vi "Lockin_Vsg.vi"(8 "error in (no error)":errorcluster, 11 "Transport":refnum<class "SMO.Transport.lvclass">) -> (0 "error out":errorcluster, 3 "Transport out":refnum<class "SMO.Transport.lvclass">)   [LabVIEW 2019, in "SMO.Transport.lvclass"]
uses:
  SMO.Transport.lvclass
  <userlib>/LevyLab/Lockin-Multichannel/Instrument.Lockin/Instrument.Lockin.lvclass
  <userlib>/LevyLab/Instrument Framework/Instrument Types/Cryostat/Instrument.Cryostat.lvclass
  Control Experiment/Control Experiment.lvclass
  <userlib>/LevyLab/Krohn Hite 7008/Instrument.KH7008.lvclass
  Control Experiment/Typedefs/Instruments--cluster.ctl
  <userlib>/LevyLab/Instrument Framework/Instrument Types/VSource/Instrument.VSource.lvclass
  <userlib>/LevyLab/Instrument Framework/Instrument Types/VNA/Instrument.VNA.lvclass
  <userlib>/LevyLab/Instrument Framework/Instrument Types/Strain/Instrument.Strain.lvclass
  <userlib>/LevyLab/Instrument Framework/Instrument Types/CBridge/Instrument.CBridge.lvclass
  <userlib>/LevyLab/Instrument Framework/Instrument Types/Delay Line/Instrument.DelayLine.lvclass
panel:
  in  "Tab Control":enum32{"lockin/SG Control", "Data", "Other"}(tab)=enum."Data"
  out "elapsed time (s)":u32=1660
  in  "Side Gate Channel(s)":i32[](array[numeric])=[21]
  in  "Vmax (end)":dbl=5.0 format="%#_3p"
  in  "Vmin (start)":dbl=-5.0 format="%#_3p"
  in  "dV":dbl=0.025 format="%#_3p"
  in  "Experiment Comments":string="Vbg sweep from  0V to 100V to  -100V to 0V in steps of 0.5V\n\nstripe device:\n\nI+: 11,12,13, current mode, gain: 1000x, shunt resistor : 5kohm \nlead 12: Vac: 125uV, 7Hz, Vdc= 0mV\ndV1: 11-12 voltage mode, gain: 10x, shunt resistor : open \nVbg: 26, 1Gohm resistor\n\nhash device:\n\nI+: 16,17 current mode, gain: 1000x, shunt resistor : 5kohm \nlead 17: Vac:  5mV, 7Hz, Vdc= 0mV\n##lead 20, voltage mode, gain: 10x, shunt resistor : open \ndV1: 16-17 voltage mode, gain: 10x, shunt resistor : open \n##dV1: 16-20 voltage mode, gain: 10x, shunt resistor : open \nVbg: 26, 1Gohm resistor\n\nIn plane gates:\n3,8,15,21: 0V, 100Mohm resistors"
  in  "Experiment Folder":string="14- mega backgate sweep"
  out "T (mK)":dbl=0.001
  in  "wait after setting Vsg (ms)":u32=2000
  in  "Initial wait (ms)":u32=1000
  in  "Sweep":enum16{"Vsg", "Vbg"}(ring)
  in  "cycles (1,2,...)":i32=1 min=1 step=1
  in  "phase":dbl
  out "Field (T)":dbl=-0.0003 format="%#_13g"
  in  "function (ramp)":enum16{"Ramp", "Triangle", "Sine"}(ring)=enum."Triangle"
  in  "set \"Vsg\" to initial value?":bool
  out "time b/w points (ms)":u32=2066
  in  "stop":bool
  out "X Lockins":cluster{dbl[], dbl[]}[](graph)
  out "Y Lockins":cluster{dbl[], dbl[]}[](graph)
  out "G4T":cluster{dbl[], dbl[]}[](graph)
  # "*** These controls are only read if this VI is the top level. If is is called from Sweep Control then the folder and comments come from Sweep Control.vi ***"
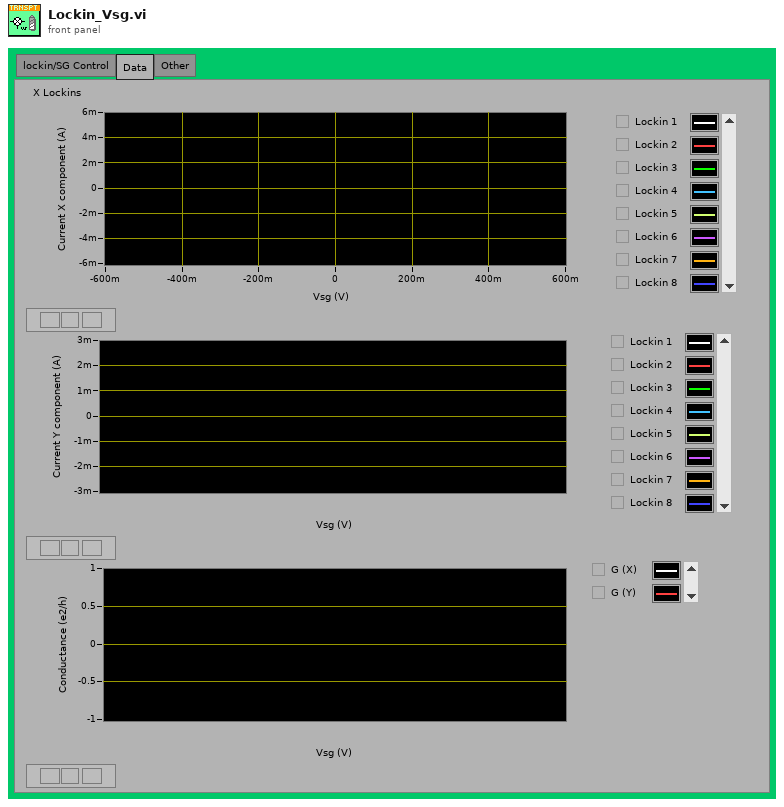
[diagram p1: front panel]
types:
  T1 = enum32{"Invalid", "Standard", "Closed", "Hidden", "Minimized", "Maximized"}
  T2 = enum32{"invalid app kind", "Development System", "Run Time System", "Student Edition", "Embedded LabVIEW", "Evaluation", "Custom"}
  T3 = typedef "Control Experiment.lvclass/Instruments--cluster.ctl" = cluster{"KH7008":refnum<class "Instrument.KH7008.lvclass">[], "Lockin":refnum<class "Instrument.Lockin.lvclass">, "Temperature":refnum<class "Instrument.Cryostat.lvclass">, "Magnet":refnum<class "Instrument.Cryostat.lvclass">, "Rotator":refnum<class "Instrument.Cryostat.lvclass">, "Level":refnum<class "Instrument.Cryostat.lvclass">, "Capacitance Bridge":refnum<class "Instrument.CBridge.lvclass">, "Delay Line":refnum<class "Instrument.DelayLine.lvclass">, "Strain Cell":refnum<class "Instrument.Strain.lvclass">, "VNA":refnum<class "Instrument.VNA.lvclass">, "Voltage Source":refnum<class "Instrument.VSource.lvclass">}
  T4 = cluster{"Core":cluster{"Current VI Reference":refnum<vi>, "Close Panel on Exit?":bool}, "Transport":refnum<class "SMO.Transport.lvclass">, "Control Experiment":refnum<class "Control Experiment.lvclass">, "Instruments":T3, "Sweep Values":dbl[], "Results (Dictionary)":cluster{"key":string, "value":dbl}[], "size":i32, "index":i32, "ms [0]":u32, "ms [i]":u32, "Execution:State":enum32{"Bad", "Idle", "Run top level", "Running"}}
  T5 = enum32{"Bad", "Idle", "Run top level", "Running"}
  T6 = cluster{"Current VI Reference":refnum<vi>, "Close Panel on Exit?":bool}
  T7 = cluster{"I-":i32, "I+":i32, "V1-":i32, "V1+":i32, "I2-":i32, "I2+":i32, "V2-":i32, "V2+":i32}
  T8 = typedef "Instrument.DAQ.lvclass/AO.Channel--Cluster--Array.ctl" = T9[]
  T9 = typedef "Instrument.DAQ.lvclass/AO.Channel--Cluster.ctl" = cluster{"Enable?":bool, "Channel":i32, "Amplitude":dbl, "Offset":dbl, "Frequency":dbl, "Phase":dbl, "Function":T10, "Sweeping?":bool}
  T10 = typedef "Instrument.DAQ.lvclass/AO.Channel.Function--Enum.ctl" = enum16{"Sine", "Triangle", "Square"}
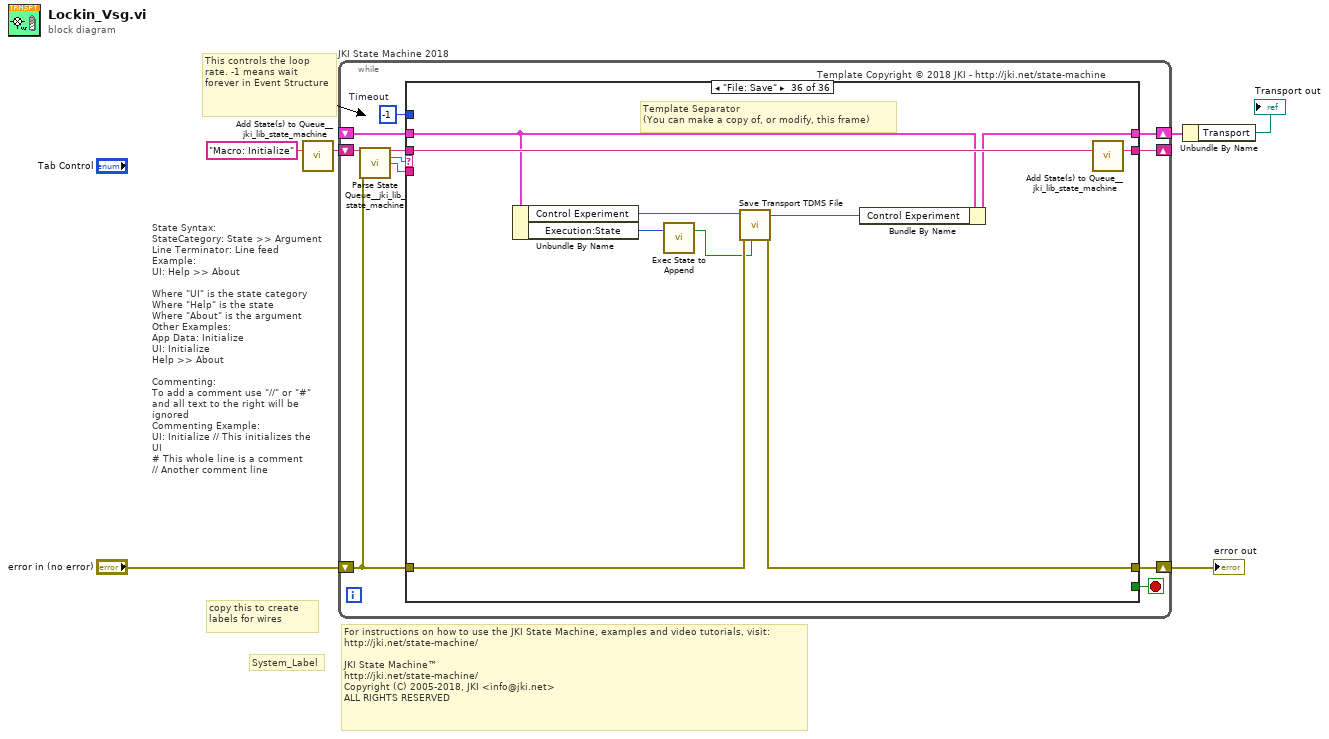
[diagram p0: block diagram]
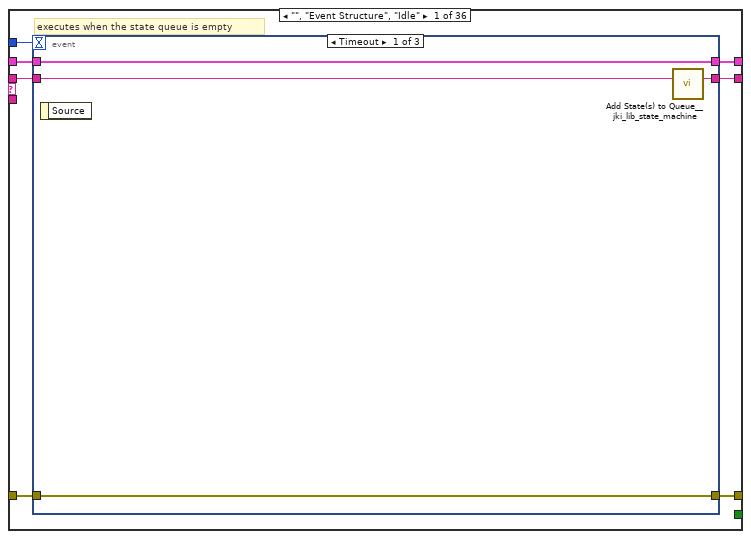
[diagram p2: hidden frame]
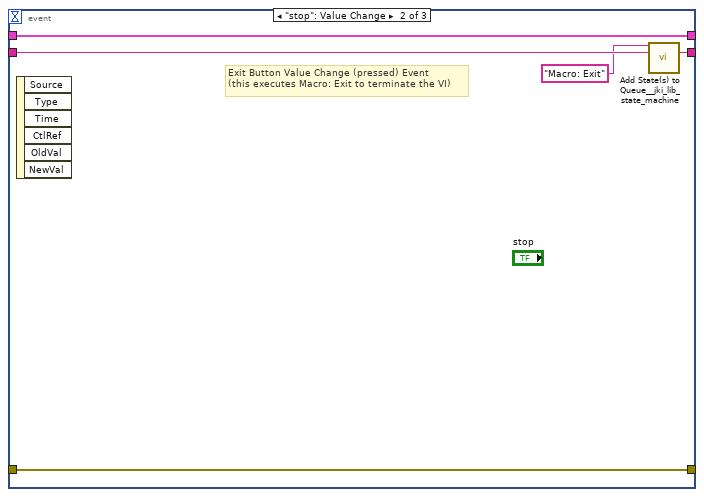
[diagram p3: hidden frame]
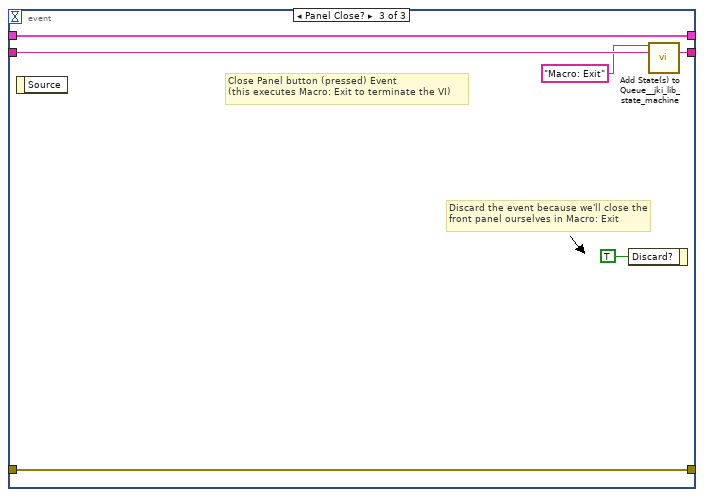
[diagram p4: hidden frame]
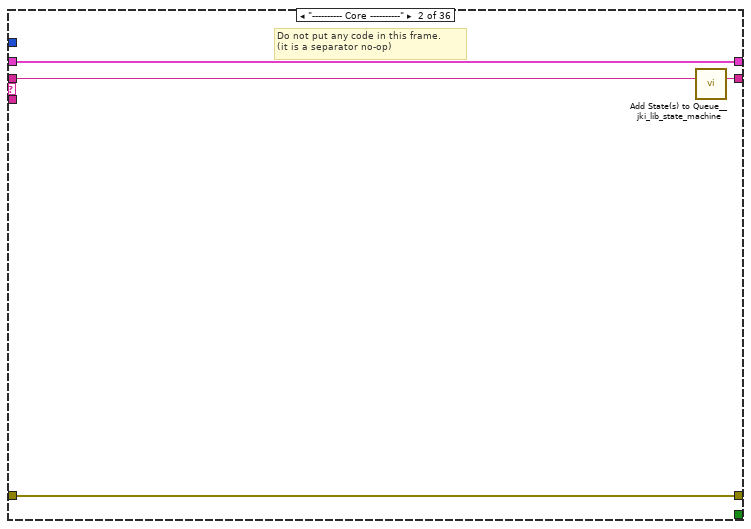
[diagram p5: hidden frame]
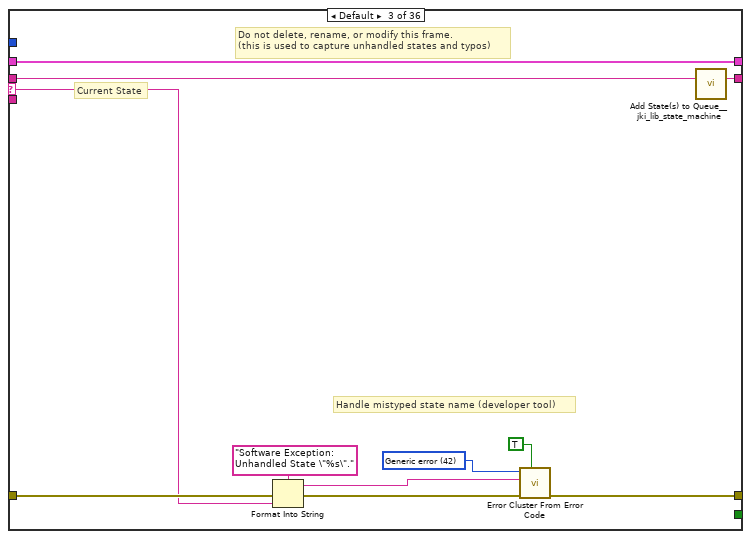
[diagram p6: hidden frame]
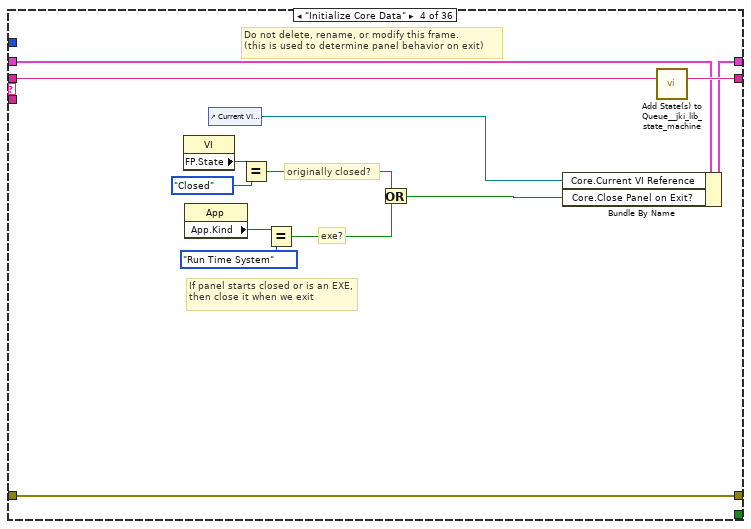
[diagram p7: hidden frame]
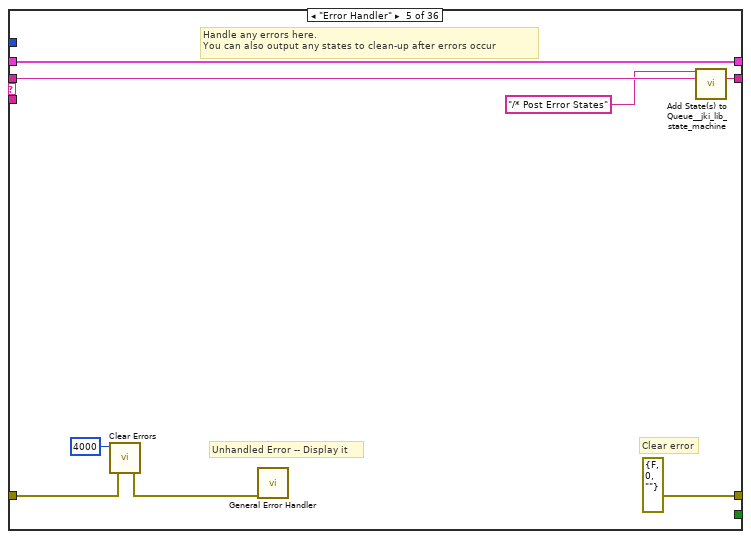
[diagram p8: hidden frame]
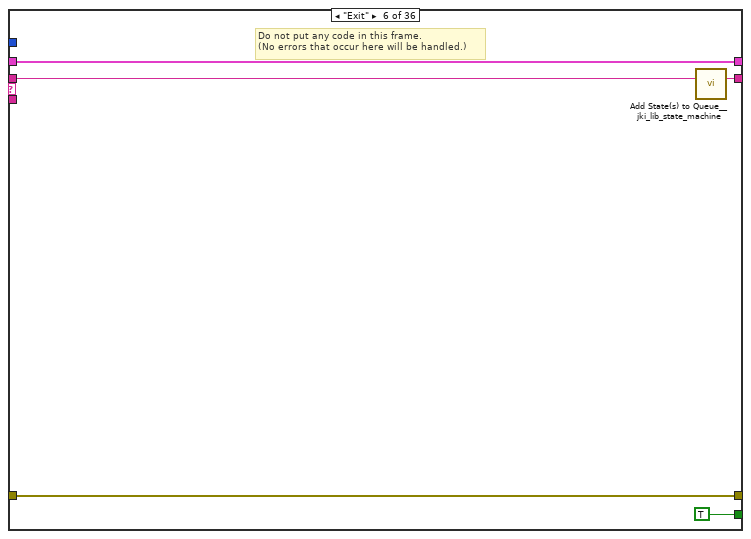
[diagram p9: hidden frame]
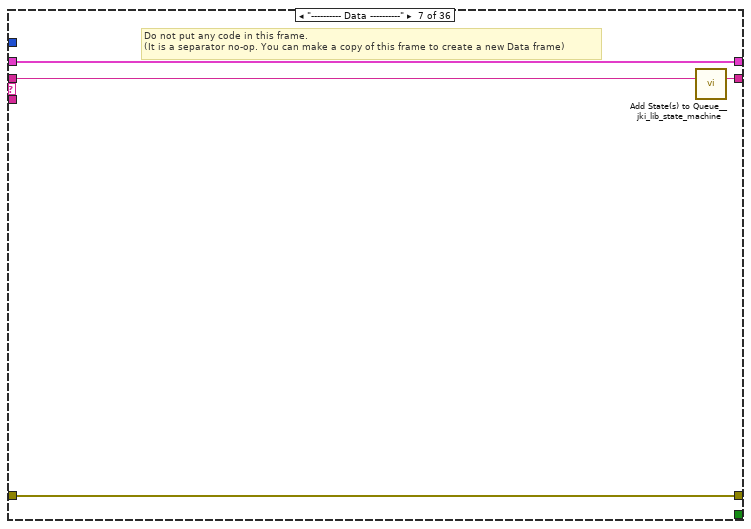
[diagram p10: hidden frame]
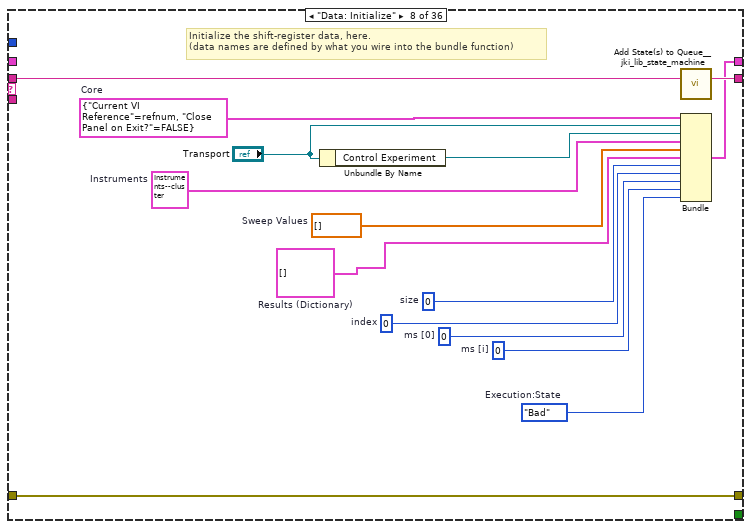
[diagram p11: hidden frame]
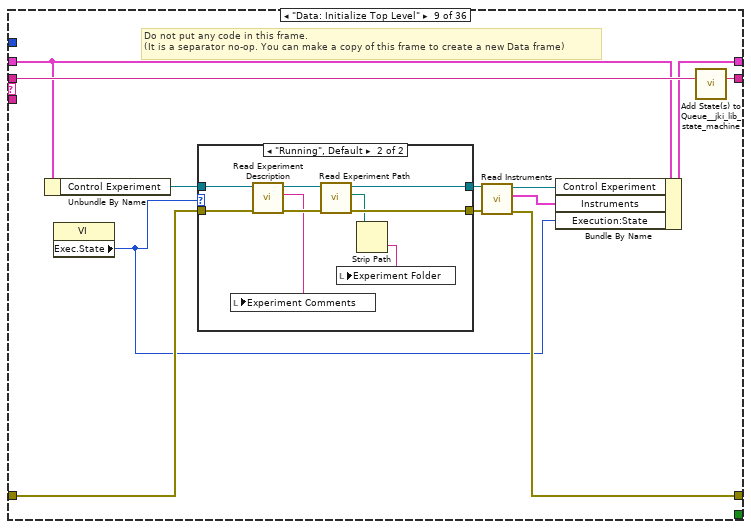
[diagram p12: hidden frame]
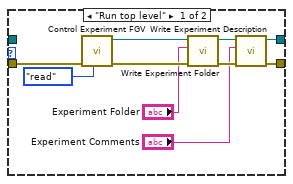
[diagram p13: hidden frame]
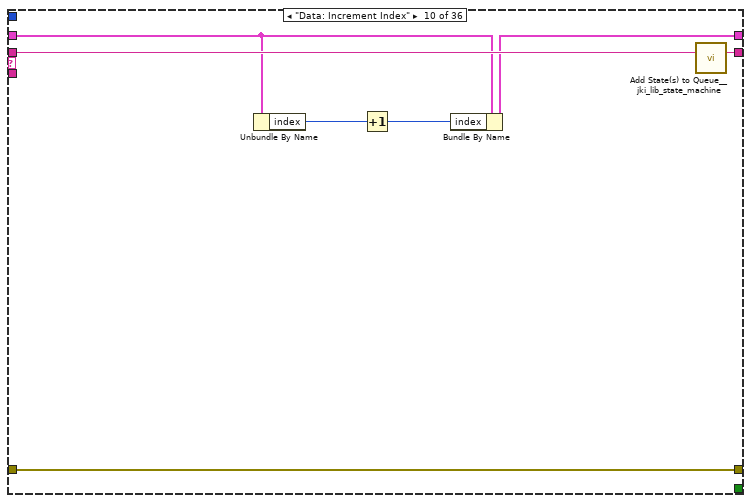
[diagram p14: hidden frame]
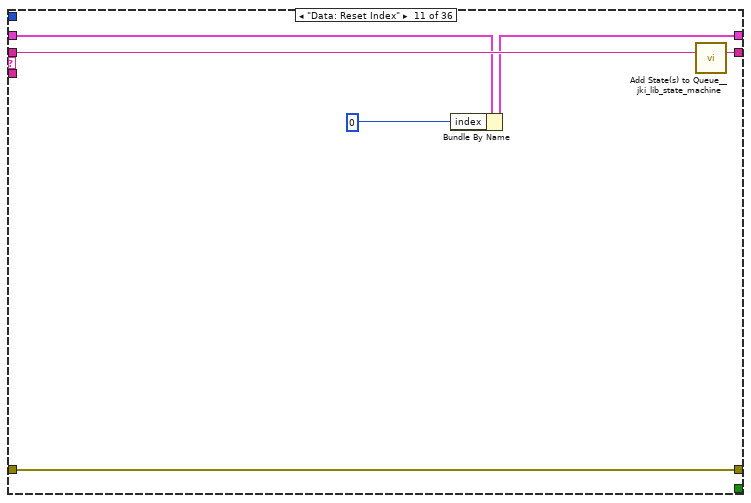
[diagram p15: hidden frame]
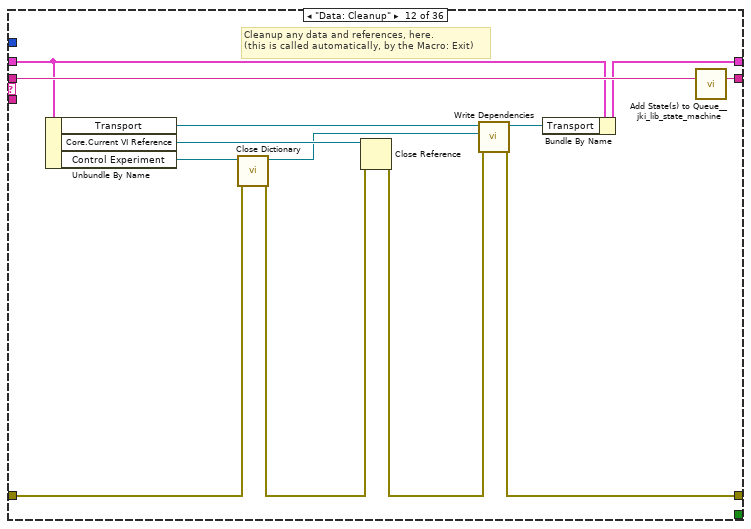
[diagram p16: hidden frame]
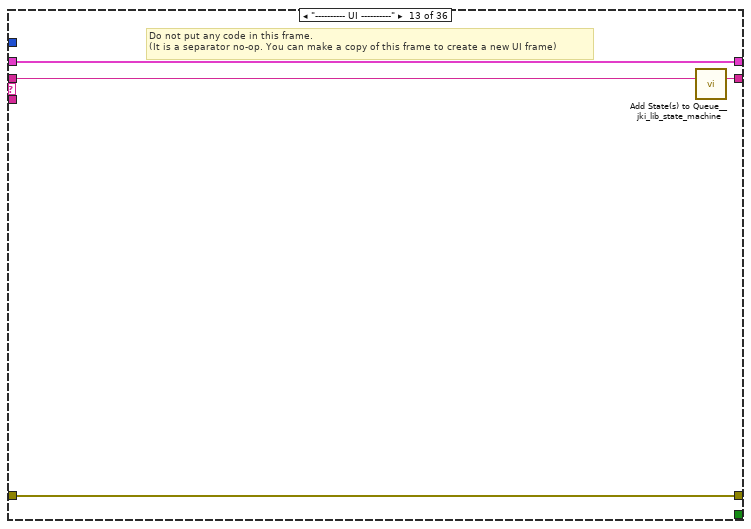
[diagram p17: hidden frame]
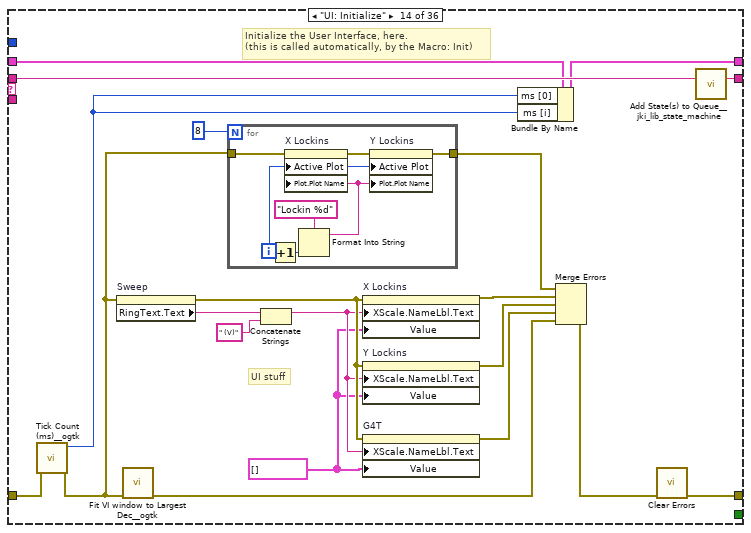
[diagram p18: hidden frame]
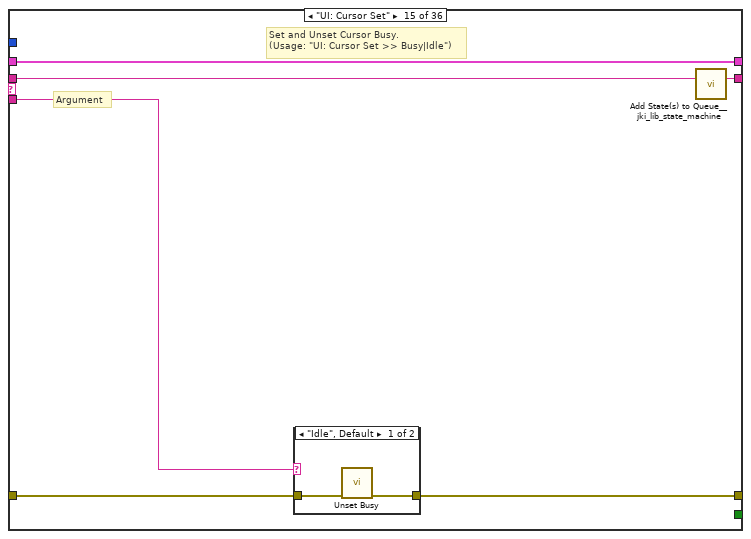
[diagram p19: hidden frame]
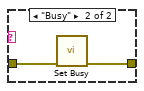
[diagram p20: hidden frame]
diagram:
  # "For instructions on how to use the JKI State Machine, examples and video tutorials, visit:\nhttp://jki.net/state-machine/\n\nJKI State Machine™\nhttp://jki.net/state-machine/\nCopyright (C) 2005-2018, JKI <info@jki.net>\nALL RIGHTS RESERVED"
  # "State Syntax:\nStateCategory: State >> Argument\nLine Terminator: Line feed\nExample:\nUI: Help >> About\n\nWhere \"UI\" is the state category\nWhere \"Help\" is the state\nWhere \"About\" is the argument\nOther Examples:\nApp Data: Initialize\nUI: Initialize\nHelp >> About\n\nCommenting:\nTo add a comment use \"//\" or \"#\" and all text to the right will be ignored\nCommenting Example:\nUI: Initialize // This initializes the UI\n# This whole line is a comment\n// Another comment line"
  # "copy this to create labels for wires"
  # "This controls the loop rate. -1 means wait forever in Event Structure"
  # "System_Label"
  n1 = call <vilib>:"Add State(s) to Queue__jki_lib_state_machine.vi"("State(s) in (\"\")"="Macro: Initialize") -> ("States Out"=w6:string)  [unwired: 14 in]
  n2 = while "JKI State Machine 2018" {
    shift-right: [w10] -> w4
    shift-left: _ -> [w9]
    shift-right: [w13] -> w2
    shift-left: "error in (no error)" -> [w7]
    shift-right: [w12] -> _
    shift-left: w6 -> [w14]
    stop <- w11 stop-if-true
    w8 = -1  # Timeout
    # "Template Copyright © 2018 JKI - http://jki.net/state-machine"
    n3 = call <vilib>:"Parse State Queue__jki_lib_state_machine.vi"("State Queue"=w14, "Error In (no error)"=w7) -> ("Remaining States"=w16:string, "Current State"=w17:string, "Arguments"=w15:string)  [unwired: 11 in]
    n4 = case shown="\"File: Save\"" w17 {
      selector: w17 -> [_ _ w44 _ _ _ _ _ _ _ _ _ _ _ _ _ _ _ _ _ _ _ _ _ _ _ _ _ _ _ _ _ _ _ _ _]
      tunnel: w16 -> [w24 w43 w48 w67 w75 w80 w84 w99 w111 w137 w143 w156 w160 w180 w193 w216 w229 w236 w305 w310 w332 w342 w346 w370 w382 w389 w401 w435 w447 w459 w471 w484 w511 w515 w519 w529]
      tunnel: w15 -> [_ _ _ _ _ _ _ _ _ _ _ _ _ _ w188 _ _ w230 _ _ _ _ _ _ _ _ _ _ _ _ _ _ _ _ _ _]
      tunnel: w9 -> [w22 w40 w46 w60 w72 w78 w81 _ w102 w131 w140 w145 w157 w164 w191 w199 w224 w232 w302 w308 w325 w339 w343 w358 w379 w385 w392 w432 w443 w456 w465 w479 w507 w512 w516 w523]
      tunnel: [w21 w41 w50 w64 errorcluster {"status"=FALSE, "code"=0, "source"=""} ("error out") w77 w82 w96 w103 w135 w141 w146 w158 w169 w189 w214 w218 w233 w303 w306 w330 w340 w344 w348 w380 w386 w395 w433 w439 w449 w461 w473 w502 w513 w517 w526] -> w13
      tunnel: w7 -> [w20 w41 w49 w64 w69 w77 w82 w96 w104 w135 w141 w152 w158 w166 w190 w214 w226 w234 w303 w306 w330 w340 w344 w355 w380 w387 w394 w433 w444 w454 w462 w482 w503 w513 w517 w525]
      tunnel: [w23 w42 w47 w66 w74 w79 w83 w98 w110 w136 w142 w155 w159 w179 w192 w215 w228 w235 w304 w309 w331 w341 w345 w369 w381 w388 w400 w434 w446 w458 w470 w483 w510 w514 w518 w528] -> w12
      tunnel: [_ _ _ _ _ TRUE _ _ _ _ _ _ _ _ _ _ _ _ _ _ _ _ _ _ _ _ _ _ _ _ _ _ _ _ _ _] -> w11
      tunnel: [w19 w40 w46 w65 w72 w78 w81 w97 w101 w134 w139 w149 w157 w163 w191 w199 w223 w232 w302 w308 w325 w339 w343 w361 w379 w385 w392 w432 w442 w455 w464 w480 w508 w512 w516 w522] -> w10
      tunnel: w8 -> [w18 _ _ _ _ _ _ _ _ _ _ _ _ _ _ _ _ _ _ _ _ _ _ _ _ _ _ _ _ _ _ _ _ _ _ _]
      frame "", "Event Structure", "Idle" {
        # "executes when the state queue is empty"
        n5 = event shown="[0] Timeout" {
          selector: _ -> [_ _ _]
          dyn-events: _ -> [_ _ _]
          timeout: w18 -> [_ _ _]
          tunnel: w24 -> [w28 w33 w39]
          tunnel: [w27 w32 w38] -> w23
          tunnel: w22 -> [w25 w30 w36]
          tunnel: [w26 w31 w37] -> w21
          tunnel: w20 -> [w26 w31 w37]
          tunnel: [w25 w30 w36] -> w19
          event Timeout {
            n6 = event-data() -> ()  [unwired: 1 in, 1 out]
            n7 = call <vilib>:"Add State(s) to Queue__jki_lib_state_machine.vi"("State(s) in (\"\")"=w28) -> ("States Out"=w27:string)  [unwired: 14 in]
          }
          event "stop": Value Change {
            # "Exit Button Value Change (pressed) Event\n(this executes Macro: Exit to terminate the VI)"
            n8 = event-data() -> ()  [unwired: 1 in, 6 out]
            n9 = call <vilib>:"Add State(s) to Queue__jki_lib_state_machine.vi"("State(s) in Front (\"\")"="Macro: Exit", "State(s) in (\"\")"=w33) -> ("States Out"=w32:string)  [unwired: 13 in]
          }
          event Panel Close? {
            # "Discard the event because we'll close the front panel ourselves in Macro: Exit"
            # "Close Panel button (pressed) Event\n(this executes Macro: Exit to terminate the VI)"
            n10 = event-data() -> ()  [unwired: 1 in, 1 out]
            n11 = event-data("Discard?"=TRUE) -> ()  [unwired: 1 in, 1 out]
            n12 = call <vilib>:"Add State(s) to Queue__jki_lib_state_machine.vi"("State(s) in Front (\"\")"="Macro: Exit", "State(s) in (\"\")"=w39) -> ("States Out"=w38:string)  [unwired: 13 in]
          }
        }
      }
      frame "---------- Core ----------" {
        # "Do not put any code in this frame.\n(it is a separator no-op)"
        n13 = call <vilib>:"Add State(s) to Queue__jki_lib_state_machine.vi"("State(s) in (\"\")"=w43) -> ("States Out"=w42:string)  [unwired: 14 in]
      }
      frame Default {
        w53 = 42 items=["No error", "Argument error", "Memory is full", "Out of zone", "End of file", "File already open", "Generic file I/O error", "File not found", "File permission error", "Disk is full", "Duplicate path", "Too many files open", "System feature not enabled", "Resource file not found", "Cannot add resource", "Resource not found", "Image not found", "Image memory error", "Pen does not exist", "Config type invalid", "Config token not found", "Config parse error", "Config memory error", "Bad external code format", "Bad external code offset", "External code not present", "Null window", "Destroy window error", "Null menu", "Print aborted", "Bad print record", "Print driver error", "Windows error during printing", "Memory error during printing", "Print dialog error", "Generic print error", "Invalid device refnum", "Device not found", "Device parameter error", "Device unit error", "Cannot open device", "Device call aborted", "Generic error", "Cancelled by user", "Object ID too low", "Object ID too high", "Object not in heap", "Unknown heap", "Unknown object (invalid DefProc)", "Unknown object (DefProc not in table)", "Message out of range", "Invalid (null) method", "Unknown message", "Manager call not supported", "Bad address", "Network operation in progress", "Network operation timed out", "Connection is busy", "Network attribute not supported", "Network error", "Address in use", "System out of memory", "Connection aborted", "Connection refused", "Not connected", "Already connected", "Connection closed", "Initialization error (interapplication manager)", "Bad occurrence", "Wait on unbound occurrence handler", "Occurrence queue overflow", "Datalog type conflict", "Unused", "Unrecognized type (interapplication manager)", "Memory corrupt", "Failed to make temporary DLL", "Old CIN version", "Drag socket not found", "Failed to load drop-object", "Failed to register OLE object", "Failed to release OLE object", "Format specifier type mismatch", "Unknown format specifier", "Too few format specifiers", "Too many format specifiers", "Scan failed", "Newer CIN version", "Error converting to variant", "Runtime menu error", "Password tampered", "Variant attribute not found", "Incompatible variant data type", "Event data is not available", "Event Store is not present", "Occurrence is not found", "Event Queue is not created", "Event info is not available", "Refnum passed is NULL", "Error retrieving Class GUID", "Error retrieving CoClass GUID", "Error retrieving TypeLib GUID.", "Bad built application magic bytes.", "Specific driver is different from the specific driver associated with the Logical Name.", "There is no session opened to the class driver.", "Max Error", "MAX - Error with config objects", "MAX - Error loading configuration", "MAX - Group not supported"]
        # "Current State"
        # "Do not delete, rename, or modify this frame.\n(this is used to capture unhandled states and typos)"
        # "Handle mistyped state name (developer tool)"
        n14 = Format Into String(format string="Software Exception: Unhandled State \"%s\"." ("message"), error in=w49, w44) -> (resulting string=w52:string, error out=w51:errorcluster)  [unwired: 1 in]
        n15 = call <vilib>:"Error Cluster From Error Code.vi"("show call chain? (False)"=TRUE, "error in (no error)"=w51, "error message (\"\")"=w52, "error code (0)"=w53) -> ("error out"=w50:errorcluster)  [unwired: 5 in]
        n16 = call <vilib>:"Add State(s) to Queue__jki_lib_state_machine.vi"("State(s) in (\"\")"=w48) -> ("States Out"=w47:string)  [unwired: 14 in]
      }
      frame "Initialize Core Data" {
        # "Do not delete, rename, or modify this frame.\n(this is used to determine panel behavior on exit)"
        # "originally closed?"
        # "exe?"
        # "If panel starts closed or is an EXE, then close it when we exit"
        n17 = property class="VI"() -> ("FP.State"=w57:T1)  [unwired: 2 in, 2 out]
        n18 = property class="App"() -> ("App.Kind"=w63:T2)  [unwired: 2 in, 2 out]
        n19 = control-ref of="Current VI Reference"() -> (w58:refnum<vi>)
        n20 = Equal?(x=w57, y=T1."Closed" ("Front Panel Window:State")) -> (x = y?=w55:bool)
        n21 = Equal?(x=w63, y=T2."Run Time System" ("Application:Kind")) -> (x = y?=w61:bool)
        n22 = Or(x=w55, y=w61) -> (x .or. y?=w59:bool)
        n23 = Bundle By Name(cluster=w60, "Core.Current VI Reference"=w58, "Core.Close Panel on Exit?"=w59) -> (w65:T4)
        n24 = call <vilib>:"Add State(s) to Queue__jki_lib_state_machine.vi"("State(s) in (\"\")"=w67) -> ("States Out"=w66:string)  [unwired: 14 in]
      }
      frame "Error Handler" {
        # "Unhandled Error -- Display it"
        # "Handle any errors here.\nYou can also output any states to clean-up after errors occur"
        # "Clear error"
        n25 = call <vilib>:"Clear Errors.vi"("error in (no error)"=w69, "specific error code to clear (0: all)"=4000) -> ("error out"=w68:errorcluster)  [unwired: 4 in, 1 out]
        n26 = call <vilib>:"General Error Handler.vi"("error in (no error)"=w68) -> ()  [unwired: 10 in, 5 out]
        n27 = call <vilib>:"Add State(s) to Queue__jki_lib_state_machine.vi"("State(s) in Front (\"\")"="/* Post Error States", "State(s) in (\"\")"=w75) -> ("States Out"=w74:string)  [unwired: 13 in]
      }
      frame "Exit" {
        # "Do not put any code in this frame.\n(No errors that occur here will be handled.)"
        n28 = call <vilib>:"Add State(s) to Queue__jki_lib_state_machine.vi"("State(s) in (\"\")"=w80) -> ("States Out"=w79:string)  [unwired: 14 in]
      }
      frame "---------- Data ----------" {
        # "Do not put any code in this frame.\n(It is a separator no-op. You can make a copy of this frame to create a new Data frame)"
        n29 = call <vilib>:"Add State(s) to Queue__jki_lib_state_machine.vi"("State(s) in (\"\")"=w84) -> ("States Out"=w83:string)  [unwired: 14 in]
      }
      frame "Data: Initialize" {
        w85 = cluster{"key":string, "value":dbl}[] []  # Results (Dictionary)
        w86 = T5."Bad"  # Execution:State
        w88 = 0  # size
        w89 = u32 0  # ms [i]
        w90 = u32 0  # ms [0]
        w91 = 0  # index
        w92 = dbl[] []  # Sweep Values
        w93 = T3 {"KH7008"=[], "Lockin"=refnum, "Temperature"=refnum, "Magnet"=refnum, "Rotator"=refnum, "Level"=refnum, "Capacitance Bridge"=refnum, "Delay Line"=refnum, "Strain Cell"=refnum, "VNA"=refnum, "Voltage Source"=refnum}  # Instruments
        w95 = T6 {"Current VI Reference"=refnum, "Close Panel on Exit?"=FALSE}  # Core
        # "Initialize the shift-register data, here.\n(data names are defined by what you wire into the bundle function)"
        n30 = Unbundle By Name("Transport") -> ("Control Experiment"=w87:refnum<class "Control Experiment.lvclass">)
        n31 = call <vilib>:"Add State(s) to Queue__jki_lib_state_machine.vi"("State(s) in (\"\")"=w99) -> ("States Out"=w98:string)  [unwired: 14 in]
        n32 = Bundle("Core"=w95, "Transport"="Transport", "Control Experiment"=w87, "Instruments"=w93, "Sweep Values"=w92, "Results (Dictionary)"=w85, "size"=w88, "index"=w91, "ms [0]"=w90, "ms [i]"=w89, "Execution:State"=w86) -> (w97:T4)  [unwired: 1 in]
      }
      frame "Data: Initialize Top Level" {
        # "Do not put any code in this frame.\n(It is a separator no-op. You can make a copy of this frame to create a new Data frame)"
        n33 = Unbundle By Name(w102) -> ("Control Experiment"=w105:refnum<class "Control Experiment.lvclass">)
        n34 = property class="VI"() -> ("Exec.State"=w100:T5)  [unwired: 2 in, 2 out]
        n35 = case shown="\"Running\", Default" w100 {
          tunnel: w104 -> [w121 w129]
          tunnel: [w116 w125] -> w106
          tunnel: [w115 w126] -> w107
          tunnel: w105 -> [_ w130]
          frame "Run top level" {
            n36 = call "Control Experiment FGV.vi"("Function"=enum16{"read", "write"}."read", "error in (no error)"=w121) -> ("error out"=w119:errorcluster, "Control Experiment.lvclass out"=w120:refnum<class "Control Experiment.lvclass">)  [unwired: 8 in]
            n37 = call "Write Experiment Folder.vi"("error in (no error)"=w119, "Experiment Folder"="Experiment Folder", "Control Experiment in"=w120) -> ("error out"=w117:errorcluster, "Control Experiment out"=w118:refnum<class "Control Experiment.lvclass">)  [unwired: 7 in]
            n38 = call "Write Experiment Description.vi"("error in (no error)"=w117, "Experiment Description"="Experiment Comments", "Control Experiment in"=w118) -> ("error out"=w116:errorcluster, "Control Experiment out"=w115:refnum<class "Control Experiment.lvclass">)  [unwired: 7 in]
          }
          frame "Running", Default {
            n39 = call "Read Experiment Description.vi"("error in (no error)"=w129, "Control Experiment in"=w130) -> ("error out"=w128:errorcluster, "Experiment Description"=w123:string, "Control Experiment out"=w127:refnum<class "Control Experiment.lvclass">)  [unwired: 7 in]
            n40 = local write "Experiment Comments"(w123) -> ()
            n41 = call "Read Experiment Path.vi"("error in (no error)"=w128, "Control Experiment in"=w127) -> ("error out"=w125:errorcluster, "Experiment Path"=w124:path, "Control Experiment out"=w126:refnum<class "Control Experiment.lvclass">)  [unwired: 7 in]
            n42 = Strip Path(path=w124) -> (name=w122:string)  [unwired: 1 out]
            n43 = local write "Experiment Folder"(w122) -> ()
          }
        }
        n44 = call "Read Instruments.vi"("error in (no error)"=w106, "Control Experiment in"=w107) -> ("error out"=w103:errorcluster, "Instruments"=w109:T3, "Control Experiment out"=w108:refnum<class "Control Experiment.lvclass">)  [unwired: 7 in]
        n45 = Bundle By Name(cluster=w102, "Control Experiment"=w108, "Instruments"=w109, "Execution:State"=w100) -> (w101:T4)
        n46 = call <vilib>:"Add State(s) to Queue__jki_lib_state_machine.vi"("State(s) in (\"\")"=w111) -> ("States Out"=w110:string)  [unwired: 14 in]
      }
      frame "Data: Increment Index" {
        n47 = Unbundle By Name(w131) -> ("index"=w133:i32)
        n48 = Increment(x=w133) -> (x+1=w132:i32)
        n49 = Bundle By Name(cluster=w131, "index"=w132) -> (w134:T4)
        n50 = call <vilib>:"Add State(s) to Queue__jki_lib_state_machine.vi"("State(s) in (\"\")"=w137) -> ("States Out"=w136:string)  [unwired: 14 in]
      }
      frame "Data: Reset Index" {
        n51 = Bundle By Name(cluster=w140, "index"=0) -> (w139:T4)
        n52 = call <vilib>:"Add State(s) to Queue__jki_lib_state_machine.vi"("State(s) in (\"\")"=w143) -> ("States Out"=w142:string)  [unwired: 14 in]
      }
      frame "Data: Cleanup" {
        # "Cleanup any data and references, here.\n(this is called automatically, by the Macro: Exit)"
        n53 = Unbundle By Name(w145) -> ("Transport"=w148:refnum<class "SMO.Transport.lvclass">, "Core.Current VI Reference"=w154:refnum<vi>, "Control Experiment"=w153:refnum<class "Control Experiment.lvclass">)
        n54 = call "Close Dictionary.vi"("error in (no error)"=w152, "Control Experiment in"=w153) -> ("error out"=w151:errorcluster, "Control Experiment out"=w144:refnum<class "Control Experiment.lvclass">)  [unwired: 8 in]
        n55 = Close Reference(reference=w154, error in (no error)=w151) -> (error out=w147:errorcluster)
        n56 = call "Write Dependencies.vi"("error in (no error)"=w147, "Control Experiment.lvclass"=w144, "Transport in"=w148) -> ("error out"=w146:errorcluster, "Transport out"=w150:refnum<class "SMO.Transport.lvclass">)  [unwired: 7 in]
        n57 = Bundle By Name(cluster=w145, "Transport"=w150) -> (w149:T4)
        n58 = call <vilib>:"Add State(s) to Queue__jki_lib_state_machine.vi"("State(s) in (\"\")"=w156) -> ("States Out"=w155:string)  [unwired: 14 in]
      }
      frame "---------- UI ----------" {
        # "Do not put any code in this frame.\n(It is a separator no-op. You can make a copy of this frame to create a new UI frame)"
        n59 = call <vilib>:"Add State(s) to Queue__jki_lib_state_machine.vi"("State(s) in (\"\")"=w160) -> ("States Out"=w159:string)  [unwired: 14 in]
      }
      frame "UI: Initialize" {
        w161 = cluster{dbl[], dbl[]}[] [] ("G4T")
        # "UI stuff"
        # "Initialize the User Interface, here.\n(this is called automatically, by the Macro: Init)"
        n60 = call <userlib>:"Tick Count (ms)__ogtk.vi"("error in (no error)"=w166) -> ("error out"=w165:errorcluster, "millisecond timer value"=w162:u32)  [unwired: 9 in]
        n61 = property on="Sweep" class="Enum (strict)"(error in=w165) -> (error out=w174:errorcluster, "RingText.Text"=w172:string)  [unwired: 1 in, 1 out]
        n62 = call <userlib>:"Fit VI window to Largest Dec__ogtk.vi"("error in (no error)"=w165) -> ("error out"=w168:errorcluster)  [unwired: 5 in, 1 out]
        n63 = for {
          N: 8 -> [_]
          tunnel: [w181] -> w175
          tunnel: w165 -> [w186]
          i -> [w184]
          n64 = Increment(x=w184) -> (x+1=w182:i32)
          n65 = Format Into String(format string="Lockin %d", w182) -> (resulting string=w185:string)  [unwired: 2 in, 1 out]
          n66 = property on="X Lockins" class="XYGraph (strict)"(error in=w186, "Active Plot"=w184, "Plot.Plot Name"=w185) -> (error out=w183:errorcluster)  [unwired: 1 in, 1 out]
          n67 = property on="Y Lockins" class="XYGraph (strict)"(error in=w183, "Active Plot"=w184, "Plot.Plot Name"=w185) -> (error out=w181:errorcluster)  [unwired: 1 in, 1 out]
        }
        n68 = Concatenate Strings(w172, " (V)" ("string")) -> (w173:string)
        n69 = property on="X Lockins" class="XYGraph (strict)"(error in=w174, "XScale.NameLbl.Text"=w173, "Value"=w161) -> (error out=w176:errorcluster)  [unwired: 1 in, 1 out]
        n70 = property on="Y Lockins" class="XYGraph (strict)"(error in=w174, "XScale.NameLbl.Text"=w173, "Value"=w161) -> (error out=w177:errorcluster)  [unwired: 1 in, 1 out]
        n71 = property on="G4T" class="XYGraph (strict)"(error in=w174, "XScale.NameLbl.Text"=w173, "Value"=w161) -> (error out=w178:errorcluster)  [unwired: 1 in, 1 out]
        n72 = Bundle By Name(cluster=w164, "ms [0]"=w162, "ms [i]"=w162) -> (w163:T4)
        n73 = Merge Errors(w175, w176, w177, w178, w168) -> (w167:errorcluster)
        n74 = call <vilib>:"Clear Errors.vi"("error in (no error)"=w167) -> ("error out"=w169:errorcluster)  [unwired: 5 in, 1 out]
        n75 = call <vilib>:"Add State(s) to Queue__jki_lib_state_machine.vi"("State(s) in (\"\")"=w180) -> ("States Out"=w179:string)  [unwired: 14 in]
      }
      frame "UI: Cursor Set" {
        # "Argument"
        # "Set and Unset Cursor Busy.\n(Usage: \"UI: Cursor Set >> Busy|Idle\")"
        n76 = case shown="\"Idle\", Default" w188 {
          tunnel: w190 -> [w195 w197]
          tunnel: [w194 w196] -> w189
          frame "Idle", Default {
            n77 = call <vilib>:"Unset Busy.vi"("error in (no error)"=w195) -> ("error out"=w194:errorcluster)  [unwired: 10 in]
          }
          frame "Busy" {
            n78 = call <vilib>:"Set Busy.vi"("error in (no error)"=w197) -> ("error out"=w196:errorcluster)  [unwired: 9 in, 1 out]
          }
        }
        n79 = call <vilib>:"Add State(s) to Queue__jki_lib_state_machine.vi"("State(s) in (\"\")"=w193) -> ("States Out"=w192:string)  [unwired: 14 in]
      }
      frame "UI: Update Graphs" {
        # "Do not put any code in this frame.\n(It is a separator no-op. You can make a copy of this frame to create a new UI frame)"
        n80 = Unbundle By Name(w199) -> ("index"=w202:i32, "Sweep Values"=w205:dbl[], "Control Experiment"=w212:refnum<class "Control Experiment.lvclass">, "Results (Dictionary)"=w198:cluster{"key":string, "value":dbl}[])
        n81 = call "Get Channel Indices.vi"("Control Experiment in"=w212) -> ("Indices"=w211:T7)  [unwired: 8 in, 2 out]
        n82 = Unbundle By Name(w211) -> ("I-"=w208:i32, "V1+"=w210:i32, "V1-"=w209:i32)
        n83 = call "Results (Dictionary) to X and Y Arrays.vi"("Results (Dictionary)"=w198) -> ("Y"=w200:dbl[], "X"=w201:dbl[])  [unwired: 9 in]
        n84 = Index Array(array=w205, index=w202) -> (element=w204:dbl)
        n85 = Equal To 0?(x=w202) -> (x = 0?=w203:bool)
        n86 = call "GraphLockin_vs_Parameter.vi"("V-"=w209, "V+"=w210, "reset?"=w203, "Current"=w208, "Parameter"=w204, "Y[ ]"=w200, "X[ ]"=w201) -> ("G(e2/h) vs Parameter"=→"G4T":cluster{"Y":dbl[], "Y":dbl[]}[], "Y vs Parameter"=→"Y Lockins":cluster{dbl[], dbl[]}[], "X vs Parameter"=→"X Lockins":cluster{dbl[], dbl[]}[])  [unwired: 1 in, 1 out]
        n87 = call <vilib>:"Add State(s) to Queue__jki_lib_state_machine.vi"("State(s) in (\"\")"=w216) -> ("States Out"=w215:string)  [unwired: 14 in]
      }
      frame "UI: Update Timer" {
        n88 = Unbundle By Name(w224) -> ("ms [0]"=w225:u32)
        n89 = call <userlib>:"Tick Count (ms)__ogtk.vi"("error in (no error)"=w226) -> ("error out"=w219:errorcluster, "millisecond timer value"=w217:u32)  [unwired: 9 in]
        n90 = Subtract(x=w217, y=w225) -> (x-y=w221:u32)
        n91 = call <userlib>:"MGI Milliseconds Since Last Call.vi"("Error In"=w219) -> ("ms"=→"time b/w points (ms)":u32, "Error Out"=w218:errorcluster)  [unwired: 5 in]
        n92 = Divide(x=w221, y=u32 1000 ("x")) -> (x/y=→"elapsed time (s)":dbl)
        n93 = Bundle By Name(cluster=w224, "ms [i]"=w217) -> (w223:T4)
        n94 = call <vilib>:"Add State(s) to Queue__jki_lib_state_machine.vi"("State(s) in (\"\")"=w229) -> ("States Out"=w228:string)  [unwired: 14 in]
      }
      frame "UI: Front Panel State" {
        # "Argument"
        # "Set Front Panel Open or Closed\n(Usage: \"UI: Front Panel State >> Open|Close\")"
        n95 = Unbundle By Name(w232) -> ("Core.Current VI Reference"=w231:refnum<vi>)
        n96 = case shown="\"Minimize\", \"Minimized\"" w230 {
          tunnel: w234 -> [w242 w257 w268 w281 w294]
          tunnel: [w244 w258 w270 w283 w296] -> w233
          tunnel: w231 -> [w243 w255 w269 w282 w295]
          frame "Open", "Standard", Default {
            w237 = T1."Standard" ("State")
            n97 = property class="VI"(reference=w243, error in=w242) -> (reference out=w240:refnum<vi>, error out=w241:errorcluster, "FP.State"=w239:T1)
            n98 = Not Equal?(x=w239, y=w237) -> (x != y?=w238:bool)
            n99 = case shown="True" w238 {
              tunnel: [w248 w250] -> w244
              tunnel: w241 -> [w247 w250]
              tunnel: w240 -> [w246 _]
              tunnel: w237 -> [w245 _]
              frame True {
                n100 = invoke class="VI" method="FP.Open"(reference=w246, error in=w247, "Activate"=TRUE, "State"=w245) -> (error out=w248:errorcluster)  [unwired: 1 in, 4 out]
              }
              frame False {
              }
            }
          }
          frame "Close", "Closed" {
            n101 = property class="VI"(reference=w255, error in=w257) -> (reference out=w254:refnum<vi>, error out=w256:errorcluster, "FP.State"=w252:T1)
            n102 = Not Equal?(x=w252, y=T1."Closed" ("Front Panel Window:State")) -> (x != y?=w251:bool)
            n103 = case shown="True" w251 {
              tunnel: [w259 w262] -> w258
              tunnel: w256 -> [w259 w261]
              tunnel: w254 -> [_ w260]
              frame False {
              }
              frame True {
                n104 = invoke class="VI" method="FP.Close"(reference=w260, error in=w261) -> (error out=w262:errorcluster)  [unwired: 1 in, 2 out]
              }
            }
          }
          frame "Hidden", "Hide" {
            w263 = T1."Hidden" ("State")
            n105 = property class="VI"(reference=w269, error in=w268) -> (reference out=w266:refnum<vi>, error out=w267:errorcluster, "FP.State"=w265:T1)
            n106 = Not Equal?(x=w265, y=w263) -> (x != y?=w264:bool)
            n107 = case shown="True" w264 {
              tunnel: [w274 w275] -> w270
              tunnel: w267 -> [w273 w275]
              tunnel: w266 -> [w272 _]
              tunnel: w263 -> [w271 _]
              frame True {
                n108 = invoke class="VI" method="FP.Open"(reference=w272, error in=w273, "State"=w271) -> (error out=w274:errorcluster)  [unwired: 2 in, 4 out]
              }
              frame False {
              }
            }
          }
          frame "Minimize", "Minimized" {
            w276 = T1."Minimized" ("State")
            n109 = property class="VI"(reference=w282, error in=w281) -> (reference out=w279:refnum<vi>, error out=w280:errorcluster, "FP.State"=w278:T1)
            n110 = Not Equal?(x=w278, y=w276) -> (x != y?=w277:bool)
            n111 = case shown="True" w277 {
              tunnel: [w287 w288] -> w283
              tunnel: w280 -> [w286 w288]
              tunnel: w279 -> [w285 _]
              tunnel: w276 -> [w284 _]
              frame True {
                n112 = invoke class="VI" method="FP.Open"(reference=w285, error in=w286, "State"=w284) -> (error out=w287:errorcluster)  [unwired: 2 in, 4 out]
              }
              frame False {
              }
            }
          }
          frame "Maximize", "Maximized" {
            w289 = T1."Maximized" ("State")
            n113 = property class="VI"(reference=w295, error in=w294) -> (reference out=w292:refnum<vi>, error out=w293:errorcluster, "FP.State"=w291:T1)
            n114 = Not Equal?(x=w291, y=w289) -> (x != y?=w290:bool)
            n115 = case shown="True" w290 {
              tunnel: [w300 w301] -> w296
              tunnel: w293 -> [w299 w301]
              tunnel: w292 -> [w298 _]
              tunnel: w289 -> [w297 _]
              frame True {
                n116 = invoke class="VI" method="FP.Open"(reference=w298, error in=w299, "State"=w297) -> (error out=w300:errorcluster)  [unwired: 2 in, 4 out]
              }
              frame False {
              }
            }
          }
        }
        n117 = call <vilib>:"Add State(s) to Queue__jki_lib_state_machine.vi"("State(s) in (\"\")"=w236) -> ("States Out"=w235:string)  [unwired: 14 in]
      }
      frame "---------- Macro ----------" {
        # "Do not put any code in this frame.\n(It is a separator no-op. You can make a copy of this frame to create a new Macro frame)"
        n118 = call <vilib>:"Add State(s) to Queue__jki_lib_state_machine.vi"("State(s) in (\"\")"=w305) -> ("States Out"=w304:string)  [unwired: 14 in]
      }
      frame "Macro: Initialize" {
        # "Initialization Macro\n(This is called once, when the VI starts)"
        n119 = call <vilib>:"Add State(s) to Queue__jki_lib_state_machine.vi"("State(s) in Front (\"\")"="Data: Initialize\nInitialize Core Data\nUI: Initialize\nUI: Front Panel State >> Open\nData: Initialize Top Level\nData: Reset Index\nMeasure: Temperature\nMeasure: Magnet\nMeasure: Capacitance\nSweep: Initialize\nMacro: Sweep", "State(s) in (\"\")"=w310) -> ("States Out"=w309:string)  [unwired: 13 in]
      }
      frame "Macro: Sweep" {
        # "stop if true"
        # "continue if true"
        # "sweep is finished"
        # "keep sweeping"
        # "Do not put any code in this frame.\n(It is a separator no-op. You can make a copy of this frame to create a new Macro frame)"
        n120 = Unbundle By Name(w325) -> ("size"=w326:i32, "index"=w329:i32)
        n121 = Decrement(x=w326) -> (x-1=w319:i32)
        n122 = local read "stop"() -> (w312:bool)
        n123 = Not Equal?(x=w319, y=w329) -> (x != y?=w314:bool)
        n124 = Not(x=w312) -> (.not. x?=w313:bool)
        n125 = And(x=w313, y=w314) -> (x .and. y?=w311:bool)
        n126 = Select(t="Data: Reset Index\nConfigure: Set" ("State(s) in Front (\"\")"), s="set \"Vsg\" to initial value?", f="" ("State(s) in Front (\"\")")) -> (s? t:f=w316:string)
        n127 = call <vilib>:"Add State(s) to Queue__jki_lib_state_machine.vi"("State(s) in Front (\"\")"="File: Save" ("State(s) in Front (\"\")"), "State(s) in (\"\")"=w316, "State(s) at Back (\"\")"="Macro: Exit" ("State(s) in Front (\"\")")) -> ("States Out"=w320:string)  [unwired: 12 in]
        n128 = Select(t="Macro: Sweep" ("State(s) in Front (\"\")"), s=w311, f=w320) -> (s? t:f=w328:string)
        n129 = call <vilib>:"Add State(s) to Queue__jki_lib_state_machine.vi"("State(s) in Front (\"\")"="Configure: Set\nConfigure: Wait\nMeasure: Lockin\nMeasure: Time\n//Measure: Temperature\nUI: Update Graphs\nUI: Update Timer\nData: Increment Index" ("State(s) in Front (\"\")"), "State(s) at Back (\"\")"=w328) -> ("States Out"=w318:string)  [unwired: 13 in]
        n130 = call <vilib>:"Add State(s) to Queue__jki_lib_state_machine.vi"("State(s) in (\"\")"=w332, "State(s) at Back (\"\")"=w318) -> ("States Out"=w331:string)  [unwired: 13 in]
      }
      frame "Macro: Exit" {
        # "Exit Macro\n(This is called once, when the VI exits)"
        n131 = Unbundle By Name(w339) -> ("Core.Close Panel on Exit?"=w338:bool)
        n132 = Select(t="UI: Front Panel State >> Close", s=w338, f="") -> (s? t:f=w335:string)
        n133 = call <vilib>:"Add State(s) to Queue__jki_lib_state_machine.vi"("State(s) in (\"\")"=w335, "State(s) at Back (\"\")"="Data: Cleanup\nExit") -> ("States Out"=w333:string)  [unwired: 13 in]
        n134 = call <vilib>:"Add State(s) to Queue__jki_lib_state_machine.vi"("State(s) in Front (\"\")"=w333, "State(s) in (\"\")"=w342) -> ("States Out"=w341:string)  [unwired: 13 in]
      }
      frame "---------- Sweep ----------" {
        # "Do not put any code in this frame.\n(It is a separator no-op. You can make a copy of this frame to create a new Macro frame)"
        n135 = call <vilib>:"Add State(s) to Queue__jki_lib_state_machine.vi"("State(s) in (\"\")"=w346) -> ("States Out"=w345:string)  [unwired: 14 in]
      }
      frame "Sweep: Initialize" {
        # "define sweep"
        # "Do not put any code in this frame.\n(It is a separator no-op. You can make a copy of this frame to create a new Macro frame)"
        n136 = Unbundle By Name(w358) -> ("Control Experiment"=w357:refnum<class "Control Experiment.lvclass">)
        n137 = local read "Side Gate Channel(s)"() -> (w350:i32[])
        n138 = call <userlib>:"Max_Min_conversion.vi"("Min"="Vmin (start)", "Max"="Vmax (end)") -> ("offset"=w363:dbl, "Amplitude"=w362:dbl)  [unwired: 8 in]
        n139 = local read "Sweep"() -> (w347:enum16{"Vsg", "Vbg"})
        n140 = call <userlib>:"Ramp.vi"("phase"="phase", "function (ramp)"="function (ramp)", "cycles (1,2,...)"="cycles (1,2,...)", "step size"="dV", "offset"=w363, "amplitude"=w362) -> ("Waveform Graph"=w359:dbl[])  [unwired: 3 in, 2 out]
        n141 = Format Into String(error in=w355, w347) -> (resulting string=w353:string, error out=w354:errorcluster)  [unwired: 2 in]
        n142 = call "Write Dictionary Element.vi"("error in (no error)"=w354, "value"=w359, "key"=w353, "Control Experiment in"=w357) -> ("error out"=w349:errorcluster, "Control Experiment out"=w352:refnum<class "Control Experiment.lvclass">)  [unwired: 6 in]
        n143 = case shown="\"Vsg\", Default" w347 {
          tunnel: w352 -> [w372 w378]
          tunnel: [w372 w377] -> w351
          tunnel: w350 -> [_ w376]
          tunnel: w349 -> [w371 w374]
          tunnel: [w371 w373] -> w348
          frame "Vbg" {
          }
          frame "Vsg", Default {
            n144 = call "Write Dictionary Element.vi"("error in (no error)"=w374, "value"=w376, "key"="Sweep Channels", "Control Experiment in"=w378) -> ("error out"=w373:errorcluster, "Control Experiment out"=w377:refnum<class "Control Experiment.lvclass">)  [unwired: 6 in]
          }
        }
        n145 = Array Size(array=w359) -> (size(s)=w356:i32)
        n146 = Bundle By Name(cluster=w358, "Sweep Values"=w359, "size"=w356, "Control Experiment"=w351) -> (w361:T4)
        n147 = call <vilib>:"Add State(s) to Queue__jki_lib_state_machine.vi"("State(s) in (\"\")"=w370) -> ("States Out"=w369:string)  [unwired: 14 in]
      }
      frame "---------- Configure ----------" {
        # "Do not put any code in this frame.\n(It is a separator no-op. You can make a copy of this frame to create a new Macro frame)"
        n148 = call <vilib>:"Add State(s) to Queue__jki_lib_state_machine.vi"("State(s) in (\"\")"=w382) -> ("States Out"=w381:string)  [unwired: 14 in]
      }
      frame "Configure: Wait" {
        # "Do not put any code in this frame.\n(It is a separator no-op. You can make a copy of this frame to create a new Macro frame)"
        n149 = Unbundle By Name(w385) -> ("index"=w384:i32)
        n150 = case shown="Default" w384 {
          tunnel: ["Initial wait (ms)" "wait after setting Vsg (ms)"] -> w383
          frame 0 {
          }
          frame Default {
          }
        }
        n151 = call <userlib>:"Wait (ms)__ogtk.vi"("error in (no error)"=w387, "milliseconds to wait"=w383) -> ("error out"=w386:errorcluster)  [unwired: 8 in, 1 out]
        n152 = call <vilib>:"Add State(s) to Queue__jki_lib_state_machine.vi"("State(s) in (\"\")"=w389) -> ("States Out"=w388:string)  [unwired: 14 in]
      }
      frame "Configure: Set" {
        # "do this instead of \nJSON file"
        # "Do not put any code in this frame.\n(It is a separator no-op. You can make a copy of this frame to create a new Macro frame)"
        n153 = Unbundle By Name(w392) -> ("Instruments.Lockin"=w399:refnum<class "Instrument.Lockin.lvclass">, "Sweep Values"=w398:dbl[], "index"=w397:i32)
        n154 = Index Array(array=w398, index=w397) -> (element=w393:dbl)
        n155 = case shown="\"Vbg\"" "Sweep" {
          tunnel: w399 -> [w403 w431]
          tunnel: w394 -> [w409 w430]
          tunnel: w393 -> [w406 w427]
          tunnel: [w408 w428] -> w395
          frame "Vsg", Default {
            n156 = call <userlib>:"getAO.vi"("Instrument.Lockin in"=w403) -> ("AOconfig"=w407:T8)  [unwired: 8 in, 2 out]
            n157 = Decrement(x="Side Gate Channel(s)") -> (x-1=w402:i32[])
            n158 = for {
              tunnel: w406 -> [w425]
              shift-right: [w421] -> w404
              shift-left: w407 -> [w423]
              tunnel: w402 -> [w422] mode=indexing
              n159 = Index Array(array=w423, index=w422) -> (element=w426:T9)
              n160 = Bundle By Name(cluster=w426, "Offset"=w425) -> (w424:T9)
              n161 = Replace Array Subset(array=w423, new element=w424, index=w422) -> (w421:T8)
            }
            n162 = disable-structure shown="Disabled" {
              disable-tunnel: w409 -> [w414 _]
              disable-tunnel: [w413 _] -> w408
              disable-tunnel: w406 -> [w412 _]
              disable-tunnel: "Side Gate Channel(s)" -> [w411 _]
              disable-tunnel: w403 -> [w410 _]
              frame Disabled {
                n163 = for {
                  tunnel: w411 -> [w416] mode=indexing
                  tunnel: w412 -> [w415]
                  tunnel: w410 -> [w420]
                  tunnel: [w417] -> _
                  tunnel: w414 -> [w419]
                  tunnel: [w418] -> w413
                  n164 = call <userlib>:"setAO_DC.vi"("error in (no error)"=w419, "DC (V)"=w415, "AO Channel"=w416, "Instrument.Lockin in"=w420) -> ("error out"=w418:errorcluster, "Instrument.Lockin out"=w417:refnum<class "Instrument.Lockin.lvclass">)  [unwired: 6 in]
                }
              }
              frame Enabled {
              }
            }
            n165 = call <userlib>:"setAO.vi"("Channels: AO"=w404, "Instrument.Lockin in"=w403) -> ()  [unwired: 8 in, 2 out]
          }
          frame "Vbg" {
            n166 = call <userlib>:"setAUX.vi"("error in (no error)"=w430, "AUX (V)"=w427, "Channel"=1, "Instrument.Lockin in"=w431) -> ("error out"=w428:errorcluster)  [unwired: 6 in, 1 out]
          }
        }
        n167 = call <vilib>:"Add State(s) to Queue__jki_lib_state_machine.vi"("State(s) in (\"\")"=w401) -> ("States Out"=w400:string)  [unwired: 14 in]
      }
      frame "---------- Measure ----------" {
        # "Template Separator\n(You can make a copy of, or modify, this frame)"
        n168 = call <vilib>:"Add State(s) to Queue__jki_lib_state_machine.vi"("State(s) in (\"\")"=w435) -> ("States Out"=w434:string)  [unwired: 14 in]
      }
      frame "Measure: Temperature" {
        # "Your code here.\n(You can make a copy of, or modify, this frame)"
        n169 = Unbundle By Name(w443) -> ("Control Experiment"=w438:refnum<class "Control Experiment.lvclass">, "Instruments.Temperature"=w445:refnum<class "Instrument.Cryostat.lvclass">)
        n170 = call-dynamic "Get Temperature.vi"("error in (no error)"=w444, "Instrument.Cryostat in"=w445) -> ("error out"=w440:errorcluster, "Temperature (K)"=w436:dbl)  [unwired: 5 in, 3 out]
        "T (mK)" <- w436
        n171 = call "Write Dictionary Element.vi"("error in (no error)"=w440, "value"=w436, "key"="Temperature", "Control Experiment in"=w438) -> ("error out"=w439:errorcluster, "Control Experiment out"=w437:refnum<class "Control Experiment.lvclass">)  [unwired: 6 in]
        n172 = Bundle By Name(cluster=w443, "Control Experiment"=w437) -> (w442:T4)
        n173 = call <vilib>:"Add State(s) to Queue__jki_lib_state_machine.vi"("State(s) in (\"\")"=w447) -> ("States Out"=w446:string)  [unwired: 14 in]
      }
      frame "Measure: Magnet" {
        # "Your code here.\n(You can make a copy of, or modify, this frame)"
        n174 = Unbundle By Name(w456) -> ("Control Experiment"=w452:refnum<class "Control Experiment.lvclass">, "Instruments.Magnet"=w457:refnum<class "Instrument.Cryostat.lvclass">)
        n175 = call-dynamic "Get Magnet.vi"("error in (no error)"=w454, "Instrument.Cryostat in"=w457) -> ("error out"=w448:errorcluster, "B Field (T)"=w451:dbl)  [unwired: 5 in, 3 out]
        "Field (T)" <- w451
        n176 = call "Write Dictionary Element.vi"("error in (no error)"=w448, "value"=w451, "key"="Magnet", "Control Experiment in"=w452) -> ("error out"=w449:errorcluster, "Control Experiment out"=w453:refnum<class "Control Experiment.lvclass">)  [unwired: 6 in]
        n177 = Bundle By Name(cluster=w456, "Control Experiment"=w453) -> (w455:T4)
        n178 = call <vilib>:"Add State(s) to Queue__jki_lib_state_machine.vi"("State(s) in (\"\")"=w459) -> ("States Out"=w458:string)  [unwired: 14 in]
      }
      frame "Measure: Capacitance" {
        # "Your code here.\n(You can make a copy of, or modify, this frame)"
        n179 = Unbundle By Name(w465) -> ("Control Experiment"=w466:refnum<class "Control Experiment.lvclass">, "Instruments.Capacitance Bridge"=w469:refnum<class "Instrument.CBridge.lvclass">)
        n180 = call-dynamic "Get Capacitance.vi"("error in (no error)"=w462, "Instrument.CBridge in"=w469) -> ("error out"=w467:errorcluster, "Capacitance (pF)"=w468:dbl)  [unwired: 7 in, 1 out]
        n181 = call "Write Dictionary Element.vi"("error in (no error)"=w467, "value"=w468, "key"="Capacitance", "Control Experiment in"=w466) -> ("error out"=w461:errorcluster, "Control Experiment out"=w463:refnum<class "Control Experiment.lvclass">)  [unwired: 6 in]
        n182 = Bundle By Name(cluster=w465, "Control Experiment"=w463) -> (w464:T4)
        n183 = call <vilib>:"Add State(s) to Queue__jki_lib_state_machine.vi"("State(s) in (\"\")"=w471) -> ("States Out"=w470:string)  [unwired: 14 in]
      }
      frame "Measure: Lockin" {
        # "Template Separator\n(You can make a copy of, or modify, this frame)"
        n184 = Unbundle By Name(w479) -> ("Control Experiment"=w476:refnum<class "Control Experiment.lvclass">, "Instruments.Lockin"=w481:refnum<class "Instrument.Lockin.lvclass">)
        n185 = call <userlib>:"waitForNewResults.vi"("error in (no error)"=w482, "Instrument.Lockin in"=w481) -> ("error out"=w474:errorcluster, "Results (Dictionary)"=w472:cluster{"key":string, "value":dbl}[])  [unwired: 7 in, 1 out]
        n186 = call "Results (Dictionary) to X and Y Arrays.vi"("Results (Dictionary)"=w472) -> ("Y"=w477:dbl[], "X"=w478:dbl[])  [unwired: 9 in]
        n187 = for {
          tunnel: w478 -> [w494] mode=indexing
          tunnel: w477 -> [w488] mode=indexing
          tunnel: w474 -> [w487]
          tunnel: [w486] -> w473
          shift-right: [w485] -> w475
          shift-left: w476 -> [w497]
          i -> [w500]
          n188 = Increment(x=w500) -> (x+1=w492:i32)
          n189 = Format Into String(format string="X%d" ("wavenames"), error in=w487, w492) -> (resulting string=w496:string, error out=w491:errorcluster)  [unwired: 1 in]
          n190 = call "Append Dictionary Element.vi"("error in (no error)"=w491, "value"=w494, "key"=w496, "Control Experiment in"=w497) -> ("error out"=w490:errorcluster, "Control Experiment out"=w493:refnum<class "Control Experiment.lvclass">)  [unwired: 6 in]
          n191 = Format Into String(format string="Y%d" ("wavenames"), error in=w490, w492) -> (resulting string=w495:string, error out=w489:errorcluster)  [unwired: 1 in]
          n192 = call "Append Dictionary Element.vi"("error in (no error)"=w489, "value"=w488, "key"=w495, "Control Experiment in"=w493) -> ("error out"=w486:errorcluster, "Control Experiment out"=w485:refnum<class "Control Experiment.lvclass">)  [unwired: 6 in]
        }
        n193 = Bundle By Name(cluster=w479, "Results (Dictionary)"=w472, "Control Experiment"=w475) -> (w480:T4)
        n194 = call <vilib>:"Add State(s) to Queue__jki_lib_state_machine.vi"("State(s) in (\"\")"=w484) -> ("States Out"=w483:string)  [unwired: 14 in]
      }
      frame "Measure: Time" {
        # "Your code here.\n(You can make a copy of, or modify, this frame)"
        n195 = Unbundle By Name(w507) -> ("Control Experiment"=w506:refnum<class "Control Experiment.lvclass">)
        n196 = Get Date/Time In Seconds() -> (seconds since 1Jan1904=w509:timestamp)
        n197 = To Double Precision Float(number=w509) -> (double precision float=w504:dbl)
        n198 = call "Write Dictionary Element.vi"("error in (no error)"=w503, "value"=w504, "key"="Time", "Control Experiment in"=w506) -> ("error out"=w502:errorcluster, "Control Experiment out"=w505:refnum<class "Control Experiment.lvclass">)  [unwired: 6 in]
        n199 = Bundle By Name(cluster=w507, "Control Experiment"=w505) -> (w508:T4)
        n200 = call <vilib>:"Add State(s) to Queue__jki_lib_state_machine.vi"("State(s) in (\"\")"=w511) -> ("States Out"=w510:string)  [unwired: 14 in]
      }
      frame "---------- File ----------" {
        # "Template Separator\n(You can make a copy of, or modify, this frame)"
        n201 = call <vilib>:"Add State(s) to Queue__jki_lib_state_machine.vi"("State(s) in (\"\")"=w515) -> ("States Out"=w514:string)  [unwired: 14 in]
      }
      frame "File: Configure" {
        # "Template Separator\n(You can make a copy of, or modify, this frame)"
        n202 = call <vilib>:"Add State(s) to Queue__jki_lib_state_machine.vi"("State(s) in (\"\")"=w519) -> ("States Out"=w518:string)  [unwired: 14 in]
      }
      frame "File: Save" {
        # "Template Separator\n(You can make a copy of, or modify, this frame)"
        n203 = Unbundle By Name(w523) -> ("Control Experiment"=w527:refnum<class "Control Experiment.lvclass">, "Execution:State"=w524:T5)
        n204 = call "Exec State to Append.vi"("Execution:State"=w524) -> ("append?"=w520:bool)  [unwired: 2 in]
        n205 = call "Save Transport TDMS File.vi"("append?"=w520, "error in (no error)"=w525, "Control Experiment in"=w527) -> ("error out"=w526:errorcluster, "Control Experiment out"=w521:refnum<class "Control Experiment.lvclass">)  [unwired: 7 in]
        n206 = Bundle By Name(cluster=w523, "Control Experiment"=w521) -> (w522:T4)
        n207 = call <vilib>:"Add State(s) to Queue__jki_lib_state_machine.vi"("State(s) in (\"\")"=w529) -> ("States Out"=w528:string)  [unwired: 14 in]
      }
    }
  }
  "error out" <- w2
  n208 = Unbundle By Name(w4) -> ("Transport"=→"Transport out":refnum<class "SMO.Transport.lvclass">)
